vi "TomCode.vi"() -> ()   [LabVIEW 2024]
panel:
  in  "Instrument":bool
  in  "Flip Hammer":bool
  out "Sliced Data":cluster{"Hit":waveform(dbl)[]}[](array[cluster])
  in  "save":bool
  in  "remove":bool
  in  "Zoom out":bool
  out "Waveform Graph":waveform(dbl)[](graph)
  in  "Load Waveform":bool
  # "Instructions:\n1. load the file\n2. click and drag on the graph to select a feature\n3. Remove gets rid of the selection\n4. Save adds the selection to a list\n5. once all are selected - save them as an instrument in your data folder"
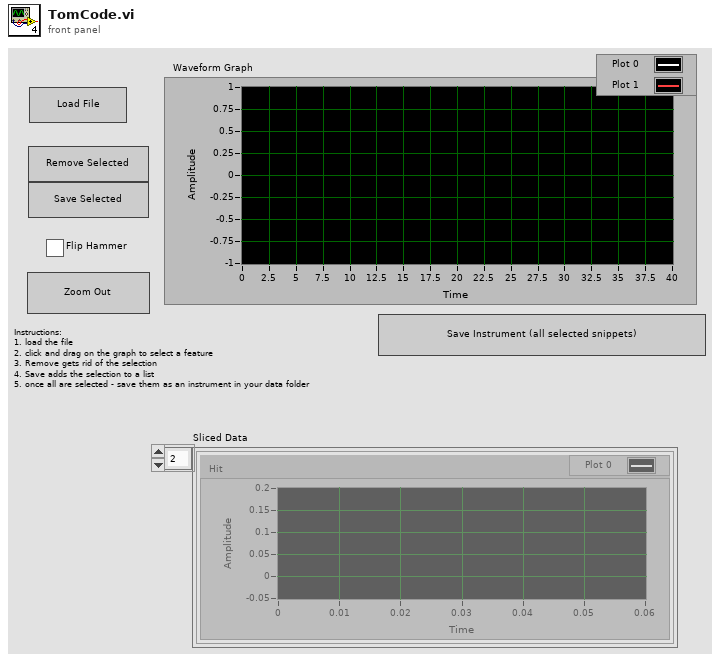
[diagram p1: front panel]
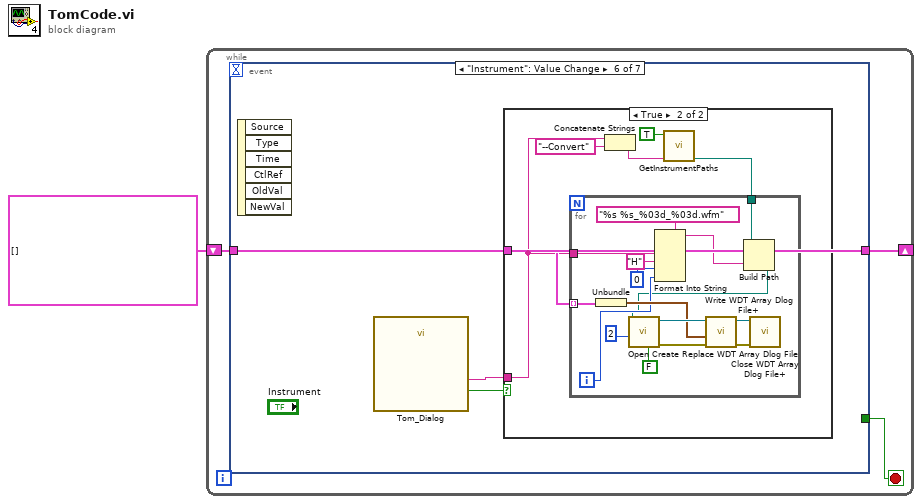
[diagram p0: block diagram]
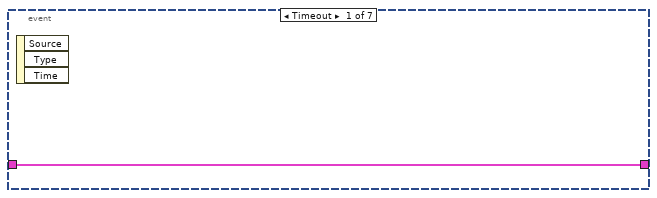
[diagram p2: hidden frame]
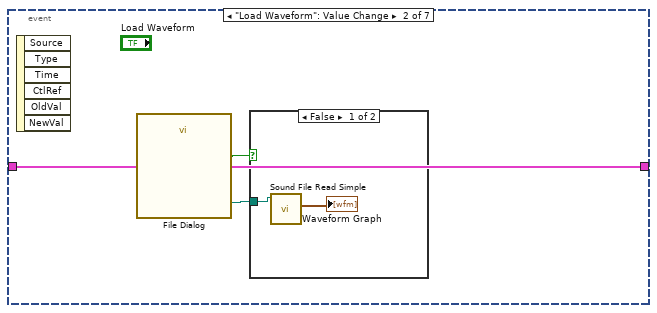
[diagram p3: hidden frame]
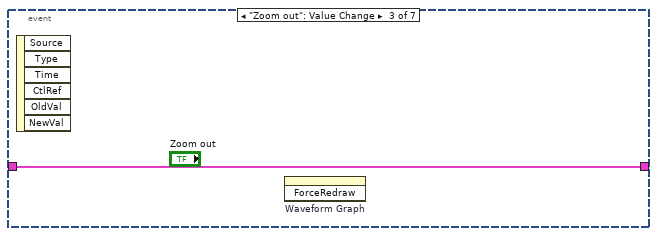
[diagram p5: hidden frame]
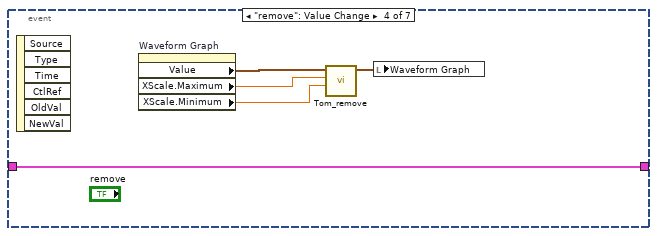
[diagram p6: hidden frame]
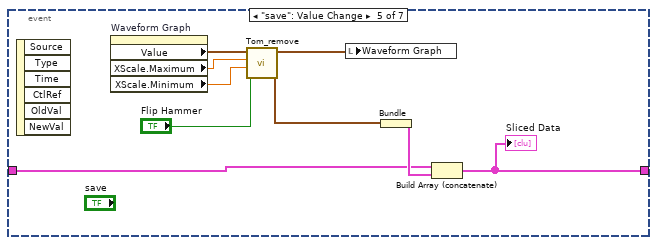
[diagram p7: hidden frame]
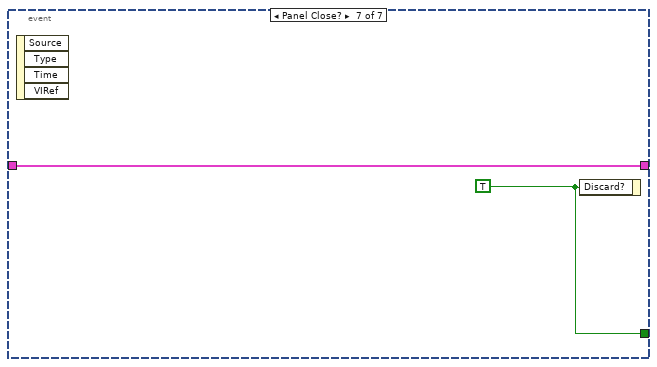
[diagram p9: hidden frame]
diagram:
  n1 = while {
    shift-right: [w3] -> _
    shift-left: cluster{"Removed":waveform(dbl)[]}[] [] -> [w2]
    stop <- w4 stop-if-true
    n2 = event shown="[5] \"Instrument\": Value Change" {
      selector: _ -> [_ _ _ _ _ _ _]
      dyn-events: _ -> [_ _ _ _ _ _ _]
      timeout: _ -> [_ _ _ _ _ _ _]
      tunnel: [_ _ _ _ _ _ w52] -> w4
      tunnel: [w5 w6 w11 w12 w19 w28 w51] -> w3
      tunnel: w2 -> [w5 w6 w11 w12 w20 w28 w51]
      event Timeout {
        n3 = event-data() -> ()  [unwired: 1 in, 3 out]
      }
      event "Load Waveform": Value Change {
        n4 = event-data() -> ()  [unwired: 1 in, 6 out]
        n5 = call "File Dialog"() -> ("selected path"=w8:path, "cancelled"=w7:bool)  [unwired: 12 in, 2 out]
        n6 = case shown="False" w7 {
          tunnel: w8 -> [w9 _]
          frame False {
            n7 = call <vilib>:"Sound File Read Simple.vi"("path"=w9) -> ("data"=→"Waveform Graph":waveform(dbl)[])  [unwired: 7 in, 3 out]
          }
          frame True {
          }
        }
      }
      event "Zoom out": Value Change {
        n8 = event-data() -> ()  [unwired: 1 in, 6 out]
        n9 = invoke on="Waveform Graph" class="WFGraph (strict)" method="ForceRedraw"() -> ()  [unwired: 3 in, 3 out]
      }
      event "remove": Value Change {
        n10 = event-data() -> ()  [unwired: 1 in, 6 out]
        n11 = property on="Waveform Graph" class="WFGraph (strict)"() -> ("Value"=w13:waveform(dbl)[], "XScale.Maximum"=w16:dbl, "XScale.Minimum"=w15:dbl)  [unwired: 2 in, 2 out]
        n12 = call "Tom_remove.vi"("XScale.Minimum"=w15, "XScale.Maximum"=w16, "Data in"=w13) -> ("Cleaned"=w14:waveform(dbl)[])  [unwired: 7 in, 1 out]
        n13 = local write "Waveform Graph"(w14) -> ()
      }
      event "save": Value Change {
        n14 = event-data() -> ()  [unwired: 1 in, 6 out]
        n15 = property on="Waveform Graph" class="WFGraph (strict)"() -> ("Value"=w22:waveform(dbl)[], "XScale.Maximum"=w25:dbl, "XScale.Minimum"=w24:dbl)  [unwired: 2 in, 2 out]
        n16 = call "Tom_remove.vi"("Flip Hammer"="Flip Hammer", "XScale.Minimum"=w24, "XScale.Maximum"=w25, "Data in"=w22) -> ("Removed"=w17:waveform(dbl)[], "Cleaned"=w23:waveform(dbl)[])  [unwired: 6 in]
        n17 = local write "Waveform Graph"(w23) -> ()
        n18 = Bundle("Removed"=w17) -> (w21:cluster{"Removed":waveform(dbl)[]})  [unwired: 1 in]
        n19 = Build Array (concatenate)(w20, w21) -> (w19:cluster{"Removed":waveform(dbl)[]}[])
        "Sliced Data" <- w19
      }
      event "Instrument": Value Change {
        n20 = event-data() -> ()  [unwired: 1 in, 6 out]
        n21 = call "Tom_Dialog.vi"() -> ("Name out"=w26:string, "OK"=w27:bool)  [unwired: 18 in]
        n22 = case shown="True" w27 {
          tunnel: w28 -> [_ w34]
          tunnel: w26 -> [_ w32]
          frame False {
          }
          frame True {
            n23 = Concatenate Strings(w32, "--Convert" ("string")) -> (w30:string)
            n24 = call "GetInstrumentPaths.vi"("Instrument"=w30, "Build?"=TRUE) -> ("Path To Raw Folder"=w33:path)  [unwired: 5 in, 4 out]
            n25 = for {
              tunnel: w34 -> [w44] mode=indexing
              tunnel: w32 -> [w41]
              tunnel: w33 -> [w37]
              i -> [w38]
              n26 = Unbundle(w44) -> ("Removed"=w43:waveform(dbl)[])
              n27 = Format Into String(format string="%s %s_%03d_%03d.wfm", w41, "H" ("input 2"), 0 ("input 3"), w38) -> (resulting string=w36:string)  [unwired: 2 in, 1 out]
              n28 = Build Path(base path=w37, name or relative path=w36) -> (appended path=w35:path)
              n29 = call <vilib>:"Open Create Replace WDT Array Dlog File.vi"("advisory dialog? (display:T)"=FALSE, "function (open:0)"=i16 2 ("create or replace"), "file path"=w35) -> ("error out"=w47:errorcluster, "refnum"=w48:refnum<k1>)  [unwired: 5 in, 2 out]
              n30 = call <vilib>:"Write WDT Array Dlog File+.vi"("error in (no error)"=w47, "Array"=w43, "refnum"=w48) -> ("error out"=w50:errorcluster, "refnum"=w49:refnum<k1>)  [unwired: 6 in, 1 out]
              n31 = call <vilib>:"Close WDT Array Dlog File+.vi"("error in (no error)"=w50, "refnum"=w49) -> ()  [unwired: 3 in, 3 out]
            }
          }
        }
      }
      event Panel Close? {
        w52 = TRUE ("Discard?")
        n32 = event-data() -> ()  [unwired: 1 in, 4 out]
        n33 = event-data("Discard?"=w52) -> ()  [unwired: 1 in, 1 out]
      }
    }
  }
